vi "VoltajeCorte.vi"(3 "Array in":dbl[][](array[numeric])) -> (0 "Voltaje de corte":dbl, 1 "Array out":cluster{"Array":dbl[], "Array out":dbl[]}[](array[cluster]))   [LabVIEW 2017]
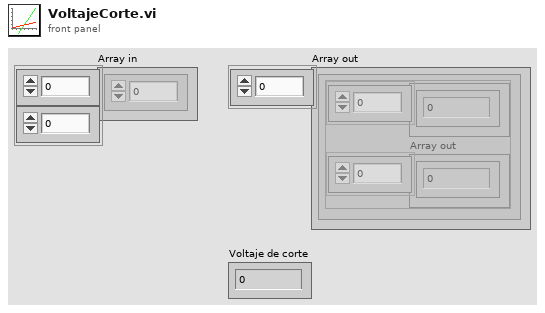
[diagram p1: front panel]
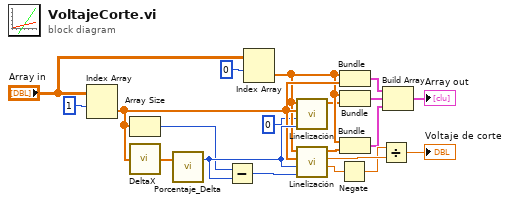
[diagram p0: block diagram]
diagram:
  n1 = Index Array(array="Array in", index (row)=1) -> (element=w13:dbl[])  [unwired: 1 in]
  n2 = Array Size(array=w13) -> (size(s)=w14:i32)
  n3 = call "DeltaX.vi"("Array in"=w13) -> ("Array out"=w6:dbl[])
  n4 = call "Porcentaje_Delta.vi"("Array in"=w6) -> ("Numeric Control"=w15:i32)  [unwired: 1 in, 1 out]
  n5 = Subtract(x=w14, y=w15) -> (x-y=w16:i32)
  n6 = Index Array(array="Array in", index (row)=0) -> (element=w10:dbl[])  [unwired: 1 in]
  n7 = call "Linelización.vi"("Longitud"=w15, "Indice"=0 ("index"), "Array Y"=w13, "Array X"=w10) -> ("Array out"=w8:dbl[])  [unwired: 5 in, 2 out]
  n8 = call "Linelización.vi"("Longitud"=w16, "Indice"=w15, "Array Y"=w13, "Array X"=w10) -> ("intercept"=w17:dbl, "slope"=w19:dbl, "Array out"=w11:dbl[])  [unwired: 5 in]
  n9 = Negate(x=w17) -> (-x=w18:dbl)
  n10 = Bundle("Array in"=w10, "Array in"=w13) -> (w5:cluster{"Array in":dbl[], "Array in":dbl[]})  [unwired: 1 in]
  n11 = Bundle("Array in"=w10, "Array out"=w8) -> (w9:cluster{"Array in":dbl[], "Array out":dbl[]})  [unwired: 1 in]
  n12 = Bundle("Array in"=w10, "Array out"=w11) -> (w12:cluster{"Array in":dbl[], "Array out":dbl[]})  [unwired: 1 in]
  n13 = Divide(x=w18, y=w19) -> (x/y=→"Voltaje de corte":dbl)
  n14 = Build Array(w5, w9, w12) -> (→"Array out":cluster{"Array in":dbl[], "Array out":dbl[]}[])
